vi "Run.vi"(8 "error in (no error)":errorcluster, 10 "sprinkler data":T2 {"Zone Indicators"."Timing" format="%#.2g"}, 11 "Controls":T6) -> (0 "error out":errorcluster, 2 "status":T1, 3 "sprinkler data out":T2 {"Zone Indicators"."Timing" format="%#.2g"})   [LabVIEW 2015]
uses:
  controls/sprinkler data.ctl
  Solution/Controls/Zone Setup.ctl
  Solution/Controls/Zone.ctl
  Solution/Controls/Zone Indicators.ctl
  controls/state.ctl
  controls/timer state.ctl
panel:
  # "Continuous"
  # "Single"
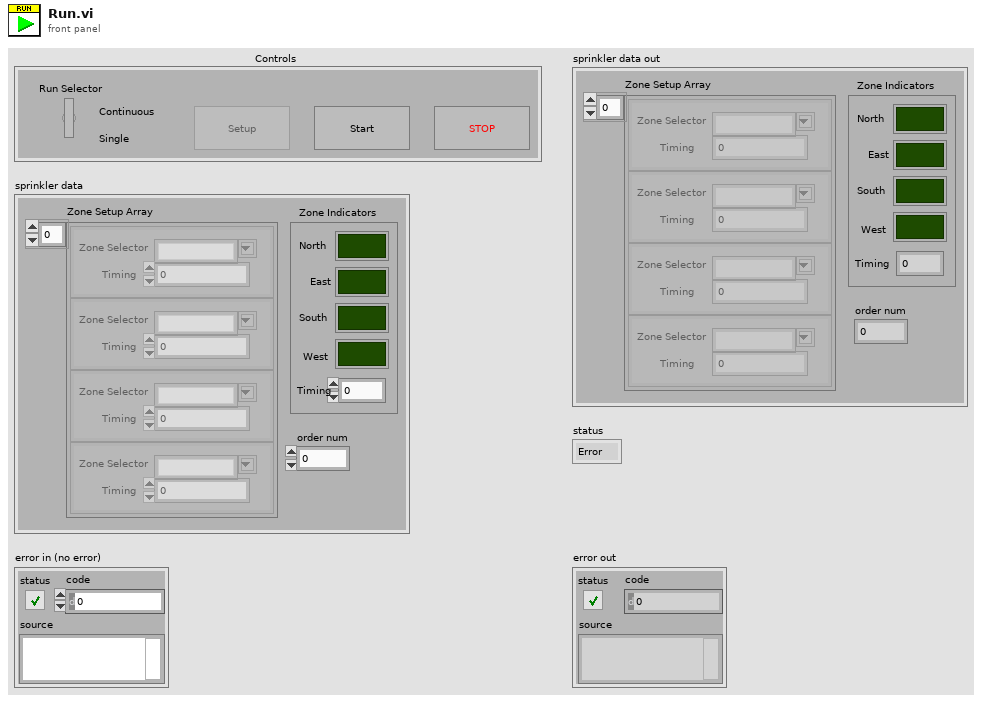
[diagram p1: front panel]
types:
  T1 = typedef "state.ctl" = enum16{"Error", "End", "Start", "Exit", "Setup", "Low pressure", "Rain", "Run", "Idle", "Initialize"}
  T2 = typedef "sprinkler data.ctl" = cluster{"Zone Setup Array":T3[], "Zone Indicators":T5, "order num":i32}
  T3 = typedef "Zone Setup.ctl" = cluster{"Zone Selector":T4, "Timing":u32}
  T4 = typedef "Zone.ctl" = string
  T5 = typedef "Zone Indicators.ctl" = cluster{"North":bool, "East":bool, "South":bool, "West":bool, "Timing":dbl}
  T6 = cluster{"Run Selector":bool, "Setup":bool, "Start":bool, "Stop":bool}
  T7 = typedef "timer state.ctl" = enum16{"Stop", "Start"}
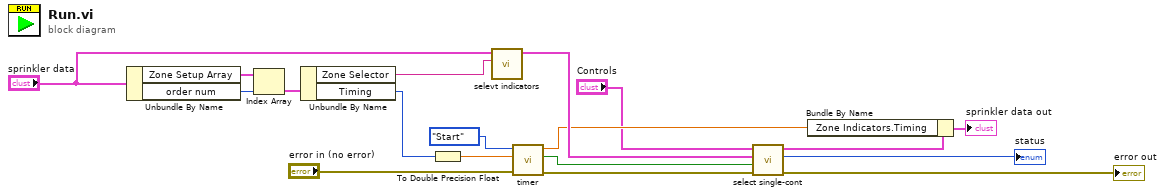
[diagram p0: block diagram]
diagram:
  n1 = Unbundle By Name("sprinkler data") -> ("Zone Setup Array"=w9:T3[], "order num"=w2:i32)
  n2 = Index Array(array=w9, index=w2) -> (element=w3:T3)
  n3 = Unbundle By Name(w3) -> ("Zone Selector"=w7:T4, "Timing"=w4:u32)
  n4 = To Double Precision Float(number=w4) -> (double precision float=w5:dbl)
  n5 = call "selevt indicators.vi"("Zone Selector"=w7, "sprinkler data in"="sprinkler data") -> ("sprinkler data out"=w14:T2)  [unwired: 9 in]
  n6 = call "timer.vi"("error in"="error in (no error)", "limit"=w5, "timer state"=timer_state."Start") -> ("error out"=w11:errorcluster, "upper limit"=w10:bool, "elapsed"=w13:dbl)  [unwired: 6 in]
  n7 = call "select single-cont.vi"("error in"=w11, "upper limit"=w10, "sprinkler data in"=w14, "Controls"="Controls") -> ("error out"=→"error out":errorcluster, "status"=→"status":T1, "sprinkler data out"=w12:T2)  [unwired: 5 in]
  n8 = Bundle By Name(cluster=w12, "Zone Indicators.Timing"=w13) -> (→"sprinkler data out":T2)
